vi "userauth_publickey.vi"() -> ()   [LabVIEW 2017]
doc: "Illustrates how to authenticate using a signing callback function."
uses:
  libssh2/libssh2_session_handshake_tcp.vi
  libssh2/libssh2_init_default.vi
  libssh2/libssh2_session_init_ex.vi
  <vilib>/Utility/tcp.llb/TCP Get Raw Net Object.vi
  libssh2/libssh2_session_handshake_socket.vi
  libssh2/libssh2.lvlib
panel:
  in  "public key":string
  in  "username":string
  in  "hostname":string="localhost"
  out "error out":errorcluster
  # "1) Insert hostname, username and public key\n2) Review the sign function (you need to implement your signing algorithm)\n3) Execute the VI"
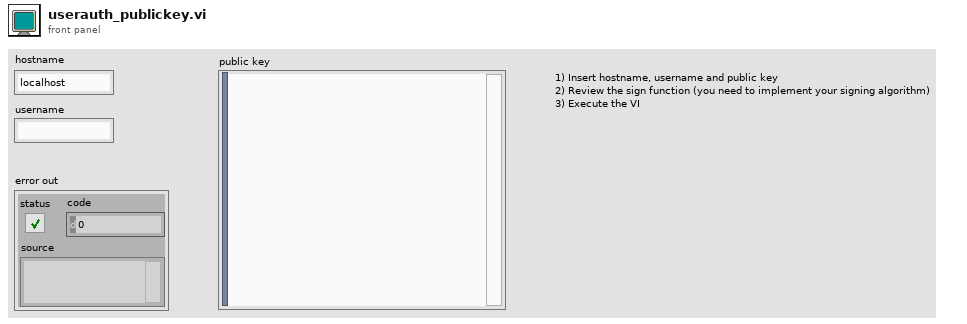
[diagram p1: front panel]
types:
  T1 = typedef "libssh2.lvlib/Session Refnum.ctl" = refnum<k1>
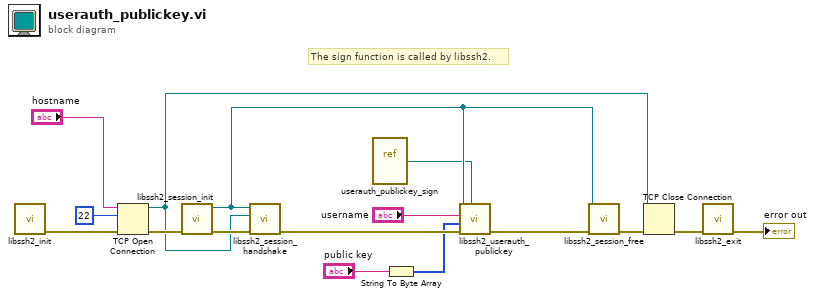
[diagram p0: block diagram]
diagram:
  # "The sign function is called by libssh2."
  n1 = call-poly "libssh2_init.vi"() -> ("error out"=w16:errorcluster)  [unwired: 11 in]
  n2 = TCP Open Connection(address="hostname", remote port or service name=u16 22, error in (no error)=w16) -> (connection ID=w7:refnum<k5>, error out=w8:errorcluster)  [unwired: 2 in]
  n3 = call "libssh2_session_init.vi"("error in (no error)"=w8) -> ("error out"=w11:errorcluster, "session"=w6:T1)  [unwired: 9 in]
  n4 = call-poly "libssh2_session_handshake.vi"("error in (no error)"=w11, "tcp connection"=w7, "session"=w6) -> ("error out"=w5:errorcluster)  [unwired: 8 in]
  n5 = vi-ref "userauth_publickey_sign.vi"() -> (w1:refnum<vi>)
  n6 = String To Byte Array(string="public key") -> (unsigned byte array=w2:u8[])
  n7 = call "libssh2_userauth_publickey.vi"("sign"=w1, "error in (no error)"=w5, "public key data"=w2, "username"="username", "session"=w6) -> ("error out"=w4:errorcluster)  [unwired: 6 in]
  n8 = call "libssh2_session_free.vi"("error in (no error)"=w4, "session"=w6) -> ("error out"=w9:errorcluster)  [unwired: 9 in]
  n9 = TCP Close Connection(connection ID=w7, error in (no error)=w9) -> (error out=w13:errorcluster)  [unwired: 1 in, 1 out]
  n10 = call "libssh2_exit.vi"("error in (no error)"=w13) -> ("error out"=→"error out":errorcluster)  [unwired: 10 in]
